vi "LR-Response-time.vi"(5 "Test characteristics":T1, 7 "Response time settings":T4={"Treshold [%]"=80}, 8 "error in (no error)":errorcluster, 9 "Power in":dbl[](array[numeric]), 11 "Results in":T3) -> (0 "error out":errorcluster, 1 "Power":dbl[](array[numeric]), 3 "Results":T3, 4 "Valid?":bool)   [LabVIEW 2013, in "MaterialCharacterization.lvlib" / "MC-LaserResponse.lvclass"]
doc: "Use this template to build a VI to use as a subVI."
uses:
  MC-LaserResponse.lvclass
  Settings-response.ctl
  Test-results.ctl
  Test-characteristics.ctl
  Detectors.ctl
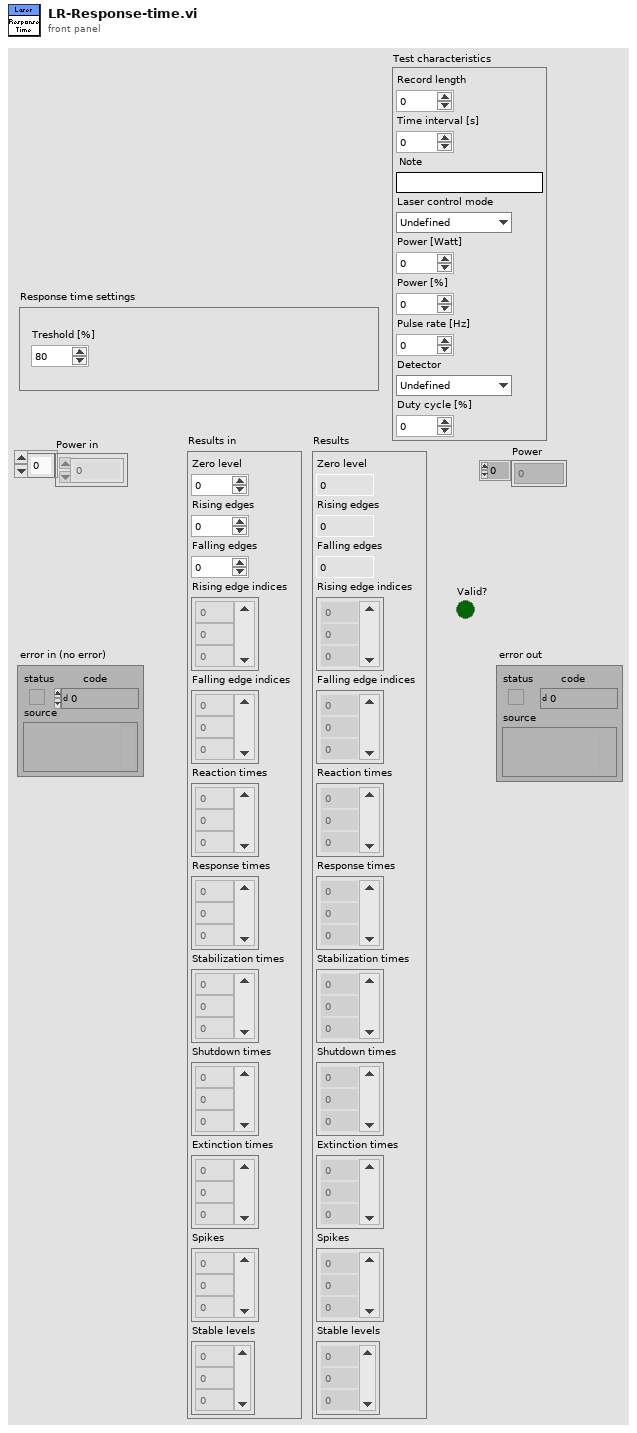
[diagram p1: front panel]
types:
  T1 = typedef "MaterialCharacterization.lvlib/MC-LaserResponse.lvclass/Test-characteristics.ctl" = cluster{"Record length":i32, "Time interval [s]":dbl, "Note":string, "Laser control mode":enum16{"Undefined", "Modulation (digital)", "Power variation (analog)"}, "Power [Watt]":dbl, "Power [%]":dbl, "Pulse rate [Hz]":dbl, "Detector":T2, "Duty cycle [%]":dbl}
  T2 = typedef "MaterialCharacterization.lvlib/MC-LaserResponse.lvclass/Detectors.ctl" = enum16{"Undefined", "DET10A", "DET10A - 2kOhm ", "PDA36A - 0dB"}
  T3 = typedef "MaterialCharacterization.lvlib/MC-LaserResponse.lvclass/Test-results.ctl" = cluster{"Zero level":dbl, "Rising edges":i32, "Falling edges":i32, "Rising edge indices":dbl[], "Falling edge indices":dbl[], "Reaction times":dbl[], "Response times":dbl[], "Stabilization times":dbl[], "Shutdown times":dbl[], "Extinction times":dbl[], "Spikes":i32[], "Stable levels":dbl[]}
  T4 = typedef "MaterialCharacterization.lvlib/MC-LaserResponse.lvclass/Settings-response.ctl" = cluster{"Treshold [%]":i32}
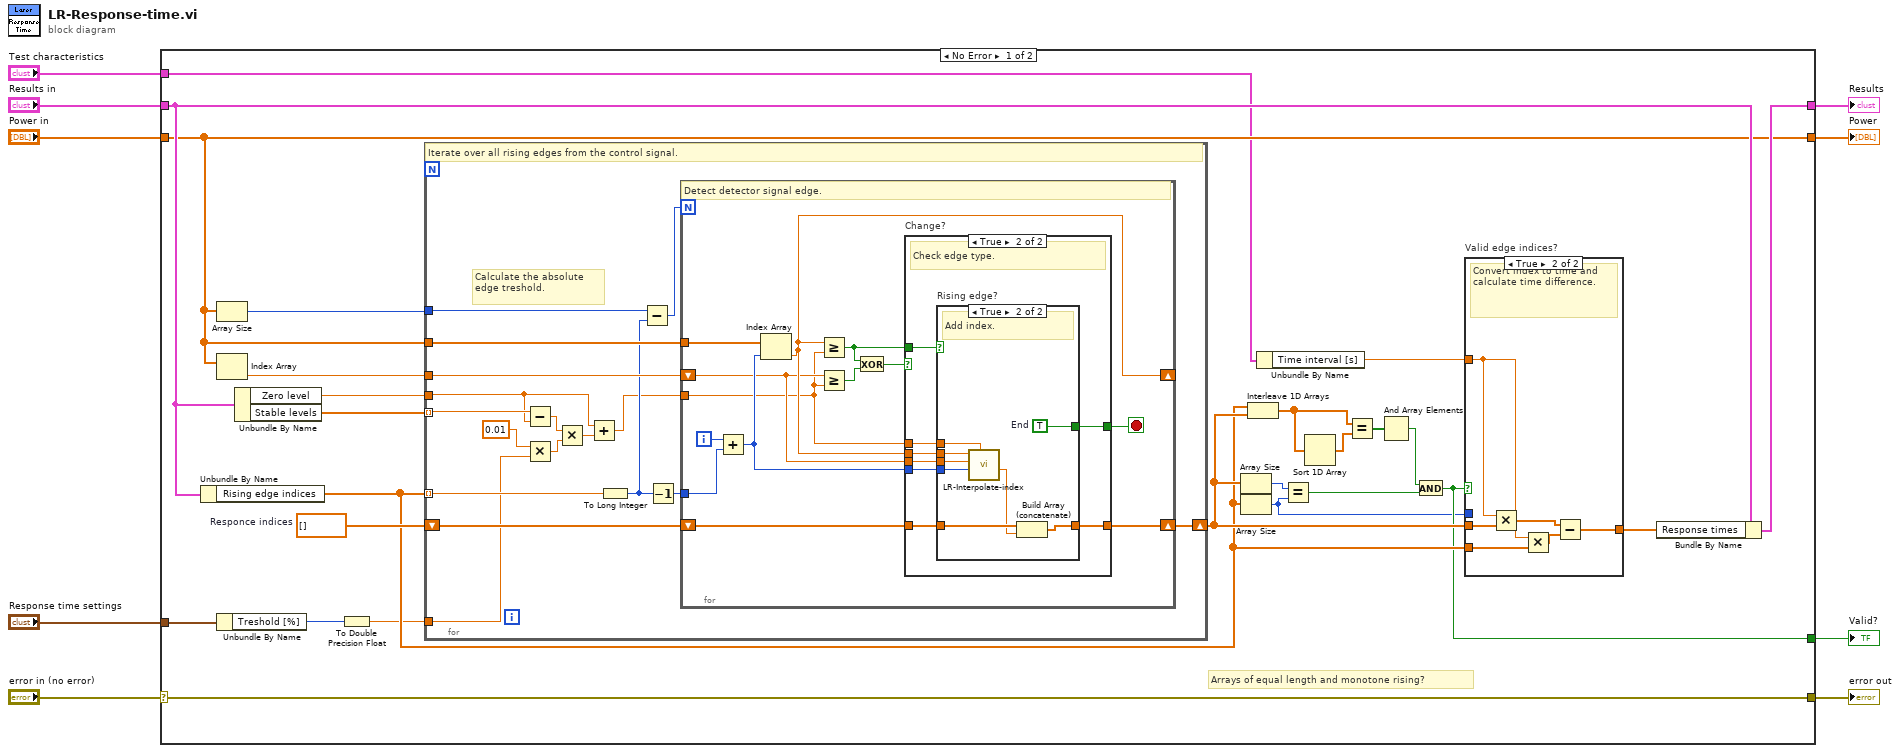
[diagram p0: block diagram]
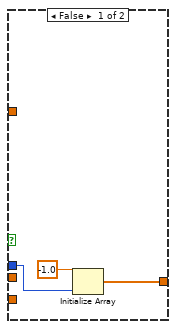
[diagram p2: hidden frame]
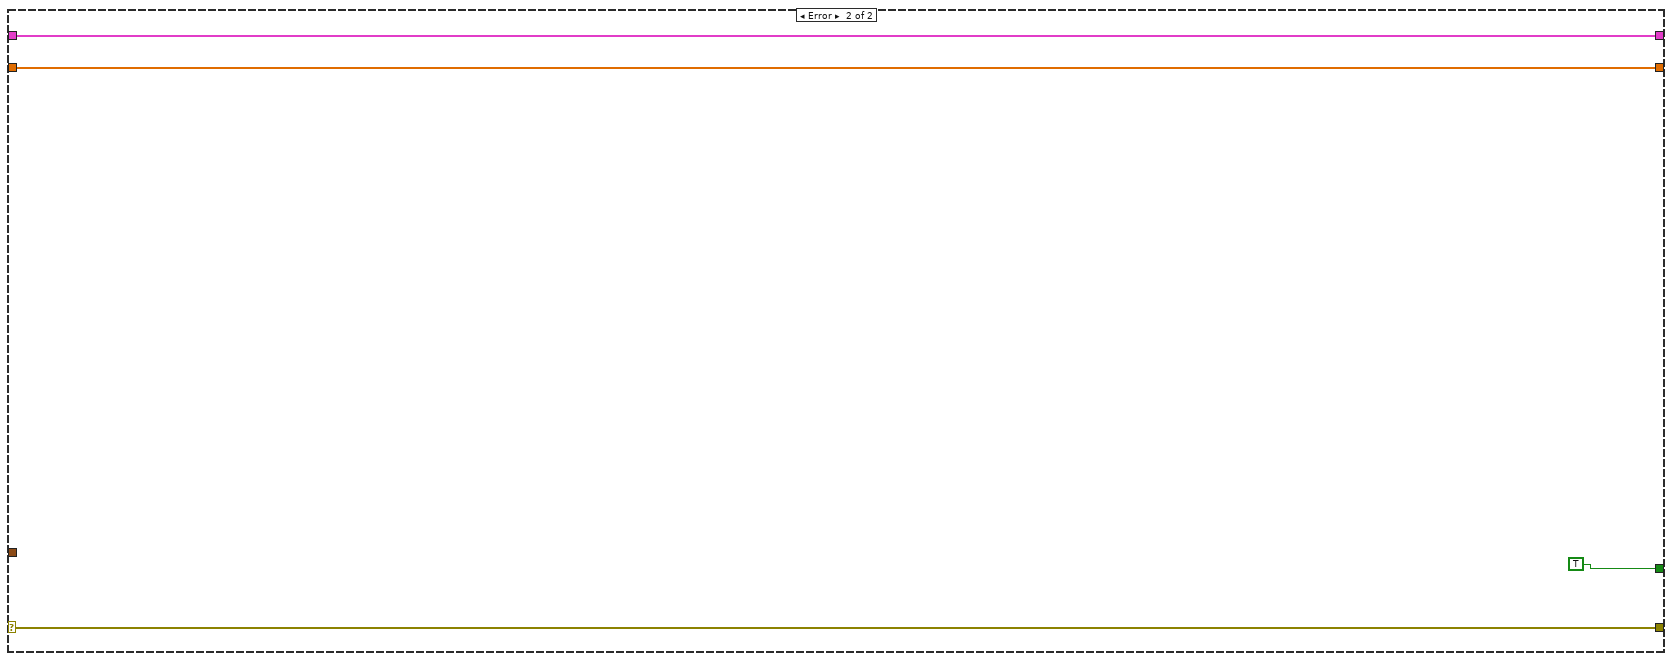
[diagram p5: hidden frame]
diagram:
  n1 = case shown="No Error" "error in (no error)" {
    selector: "error in (no error)" -> [w31 w95]
    tunnel: [w31 w95] -> w8
    tunnel: "Results in" -> [w26 w94]
    tunnel: "Response time settings" -> [w34 _]
    tunnel: [w20 TRUE] -> w7
    tunnel: [w27 w94] -> w3
    tunnel: "Power in" -> [w16 w92]
    tunnel: [w16 w92] -> w2
    tunnel: "Test characteristics" -> [w15 _]
    frame No Error {
      w32 = dbl[] []  # Responce indices
      # "Arrays of equal length and monotone rising?"
      n2 = Unbundle By Name(w26) -> ("Rising edge indices"=w21:dbl[])
      n3 = Array Size(array=w16) -> (size(s)=w18:i32)
      n4 = Index Array(array=w16) -> (element=w33:dbl)  [unwired: 1 in]
      n5 = Unbundle By Name(w34) -> ("Treshold [%]"=w11:i32)
      n6 = Unbundle By Name(w26) -> ("Zero level"=w13:dbl, "Stable levels"=w12:dbl[])
      n7 = To Double Precision Float(number=w11) -> (double precision float=w10:dbl)
      n8 = for {
        tunnel: w33 -> [w60]
        tunnel: w16 -> [w59]
        tunnel: w21 -> [w54] mode=indexing
        shift-right: [w57] -> w22
        shift-left: w32 -> [w58]
        tunnel: w18 -> [w55]
        tunnel: w13 -> [w46]
        tunnel: w12 -> [w47] mode=indexing
        tunnel: w10 -> [w44]
        # "Calculate the absolute\nedge treshold."
        # "Iterate over all rising edges from the control signal."
        n9 = Subtract(x=w47, y=w46) -> (x-y=w49:dbl)
        n10 = Multiply(x=0.01, y=w44) -> (x*y=w50:dbl)
        n11 = Multiply(x=w49, y=w50) -> (x*y=w48:dbl)
        n12 = Add(x=w46, y=w48) -> (x+y=w45:dbl)
        n13 = To Long Integer(number=w54) -> (32bit integer=w52:i32)
        n14 = Subtract(x=w55, y=w52) -> (x-y=w53:i32)
        n15 = Decrement(x=w52) -> (x-1=w56:i32)
        n16 = for {
          N: w53 -> [_]
          tunnel: w59 -> [w67]
          tunnel: w45 -> [w61]
          shift-right: [w69] -> w57
          shift-left: w58 -> [w70]
          shift-right: [w63] -> _
          shift-left: w60 -> [w62]
          tunnel: w56 -> [w66]
          i -> [w68]
          stop <- w64 stop-if-true
          # "Detect detector signal edge."
          n17 = Add(x=w68, y=w66) -> (x+y=w65:i32)
          n18 = Index Array(array=w67, index=w65) -> (element=w63:dbl)
          n19 = Greater Or Equal?(x=w63, y=w61) -> (x >= y?=w71:bool)
          n20 = Greater Or Equal?(x=w62, y=w61) -> (x >= y?=w72:bool)
          n21 = Exclusive Or(1:w72, 2:w71) -> (0:w73:bool)
          n22 = case "Change?" shown="True" w73 {
            tunnel: w71 -> [_ w82]
            tunnel: w70 -> [w74 w81]
            tunnel: w65 -> [_ w80]
            tunnel: [w74 w79] -> w69
            tunnel: [_ w78] -> w64
            tunnel: w63 -> [_ w77]
            tunnel: w62 -> [_ w76]
            tunnel: w61 -> [_ w75]
            frame False {
              # "Do nothing."
            }
            frame True {
              # "Check edge type."
              n23 = case "Rising edge?" shown="True" w82 {
                tunnel: w81 -> [w83 w91]
                tunnel: w80 -> [_ w87]
                tunnel: [w83 w90] -> w79
                tunnel: [_ w89] -> w78
                tunnel: w77 -> [_ w86]
                tunnel: w76 -> [_ w85]
                tunnel: w75 -> [_ w84]
                frame False {
                  # "Add index."
                }
                frame True {
                  w89 = TRUE  # End
                  # "Add index."
                  n24 = call "LR-Interpolate-index.vi"("Value"=w84, "Lower index"=w87, "Previous"=w85, "Current"=w86) -> ("Fractional index"=w88:dbl)  [unwired: 6 in, 1 out]
                  n25 = Build Array (concatenate)(w91, w88) -> (w90:dbl[])
                }
              }
            }
          }
        }
      }
      n26 = Array Size(array=w22) -> (size(s)=w25:i32)
      n27 = Array Size(array=w21) -> (size(s)=w17:i32)
      n28 = Interleave 1D Arrays(w21, w22) -> (w30:dbl[])
      n29 = Unbundle By Name(w15) -> ("Time interval [s]"=w14:dbl)
      n30 = Equal?(x=w25, y=w17) -> (x = y?=w23:bool)
      n31 = Sort 1D Array(array=w30) -> (sorted array=w29:dbl[])
      n32 = Equal?(x=w30, y=w29) -> (x = y?=w28:bool[])
      n33 = And Array Elements(Boolean array=w28) -> (logical AND=w24:bool)
      n34 = And(x=w24, y=w23) -> (x .and. y?=w20:bool)
      n35 = case "Valid edge indices?" shown="True" w20 {
        tunnel: w22 -> [_ w39]
        tunnel: w21 -> [_ w40]
        tunnel: [w35 w41] -> w19
        tunnel: w17 -> [w36 _]
        tunnel: w14 -> [_ w38]
        frame False {
          n36 = Initialize Array(-1.0, w36) -> (w35:dbl[])
        }
        frame True {
          # "Convert index to time and calculate time difference."
          n37 = Multiply(x=w38, y=w39) -> (x*y=w42:dbl[])
          n38 = Multiply(x=w38, y=w40) -> (x*y=w43:dbl[])
          n39 = Subtract(x=w42, y=w43) -> (x-y=w41:dbl[])
        }
      }
      n40 = Bundle By Name(cluster=w26, "Response times"=w19) -> (w27:T3)
    }
    frame Error {
    }
  }
  "error out" <- w8
  "Valid?" <- w7
  "Power" <- w2
  "Results" <- w3
